vi "SendMessageToLog.vi"(7 "Log and view ?":T1, 8 "error in (no error)":errorcluster, 9 "Criticity":T2, 10 "Message":string, 11 "EVE reference in":refnum<data-value>) -> (0 "error out":errorcluster, 3 "EVE reference out":refnum<data-value>)   [LabVIEW 2013]
uses:
  030 - EVENTS/03 - ToMessageHandlerProcess/enumMessageCriticity.ctl
  Ctrls/enumLogAndView.ctl
  001 - MAIN/Class/EVE/EVE.lvclass
  030 - EVENTS/03 - ToMessageHandlerProcess/ToMessageHandlerEvent.ctl
  001 - MAIN/Class/Messages/Messages.lvclass
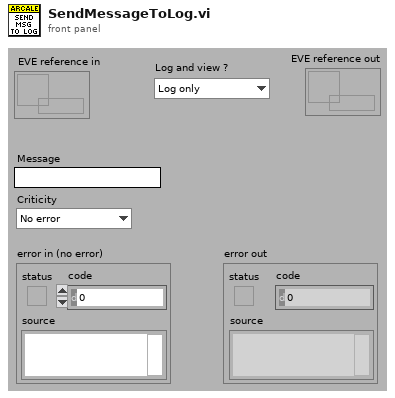
[diagram p1: front panel]
types:
  T1 = typedef "enumLogAndView.ctl" = enum16{"Log only", "Log and view"}
  T2 = typedef "enumMessageCriticity.ctl" = enum16{"No error", "Info", "Warning", "Error", "Fatal error"}
  T3 = typedef "ToMessageHandlerEvent.ctl" = cluster{"date / time":timestamp, "Criticity":T2, "Emitter":string, "Message":string}
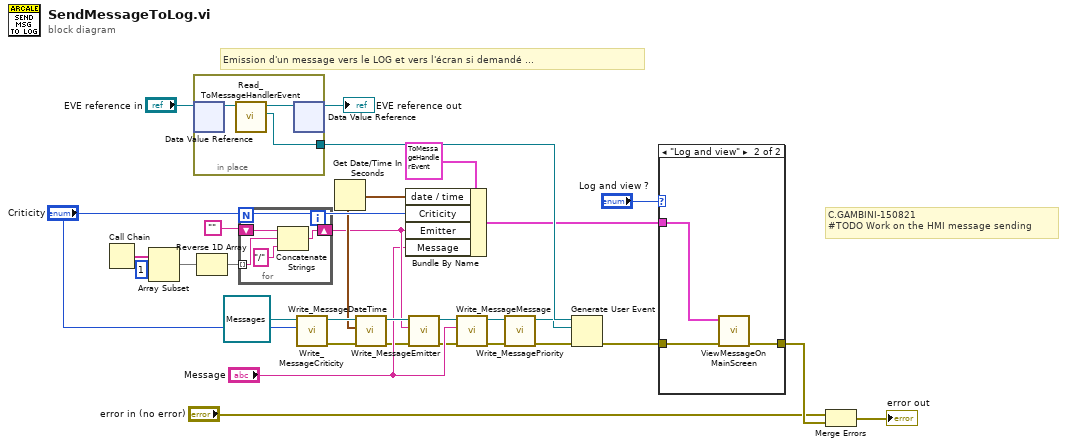
[diagram p0: block diagram]
diagram:
  # "C.GAMBINI-150821\n#TODO Work on the HMI message sending"
  # "Emission d'un message vers le LOG et vers l'écran si demandé ..."
  n1 = Call Chain() -> (call chain=w23:string[])
  n2 = Array Subset(array=w23, index=1) -> (w25:string[])  [unwired: 1 in]
  n3 = in-place {
    in-place-border: [w33] -> w30
    n4 = in-place-dvr #1("EVE reference in") -> (w32:refnum<class "EVE.lvclass">)  [unwired: 1 out]
    n5 = call-dynamic "Read_ToMessageHandlerEvent.vi"("EVE in"=w32) -> ("To message handler event"=w33:refnum<user-event>, "EVE out"=w31:refnum<class "EVE.lvclass">)  [unwired: 8 in, 1 out]
    n6 = in-place-dvr #1(w31) -> (→"EVE reference out":refnum<data-value>)  [unwired: 1 out]
  }
  n7 = Reverse 1D Array(array=w25) -> (reversed array=w22:string[])
  n8 = for {
    tunnel: w22 -> [w35] mode=indexing
    shift-right: [w37] -> w11
    shift-left: "" -> [w36]
    n9 = Concatenate Strings(w36, w35, "/" ("string")) -> (w37:string)
  }
  n10 = call-dynamic "Write_MessageCriticity.vi"("Criticity"="Criticity", "Messages in"=refnum<class "Messages.lvclass"> refnum ("Messages.lvclass")) -> ("error out"=w5:errorcluster, "Messages out"=w18:refnum<class "Messages.lvclass">)  [unwired: 8 in]
  n11 = Get Date/Time In Seconds() -> (seconds since 1Jan1904=w12:timestamp)
  n12 = call-dynamic "Write_MessageDateTime.vi"("error in (no error)"=w5, "date / time"=w12, "Messages in"=w18) -> ("error out"=w4:errorcluster, "Messages out"=w17:refnum<class "Messages.lvclass">)  [unwired: 7 in]
  n13 = Bundle By Name(cluster=T3 {"date / time"=timestamp(0 s since 1904-01-01), "Criticity"=enum."No error", "Emitter"="", "Message"=""} ("event data"), "date / time"=w12, "Criticity"="Criticity", "Emitter"=w11, "Message"="Message") -> (w27:T3)
  n14 = call-dynamic "Write_MessageEmitter.vi"("error in (no error)"=w4, "Emitter"=w11, "Messages in"=w17) -> ("error out"=w3:errorcluster, "Messages out"=w16:refnum<class "Messages.lvclass">)  [unwired: 7 in]
  n15 = call-dynamic "Write_MessageMessage.vi"("error in (no error)"=w3, "Message"="Message", "Messages in"=w16) -> ("error out"=w2:errorcluster, "Messages out"=w15:refnum<class "Messages.lvclass">)  [unwired: 7 in]
  n16 = call-dynamic "Write_MessagePriority.vi"("error in (no error)"=w2, "Messages in"=w15) -> ("error out"=w1:errorcluster, "Messages out"=w9:refnum<class "Messages.lvclass">)  [unwired: 8 in]
  n17 = Generate User Event(user event=w30, event data cluster=w9, error in=w1) -> (error out=w28:errorcluster)  [unwired: 1 in, 1 out]
  n18 = case shown="\"Log and view\"" "Log and view ?" {
    tunnel: w28 -> [w38 w41]
    tunnel: [w38 w40] -> w20
    tunnel: w27 -> [_ w39]
    frame "Log only", Default {
    }
    frame "Log and view" {
      n19 = call "ViewMessageOnMainScreen.vi"("error in (no error)"=w41, "Message"=w39) -> ("error out"=w40:errorcluster)  [unwired: 9 in]
    }
  }
  n20 = Merge Errors("error in (no error)", w20) -> (→"error out":errorcluster)
